vi "Variable@Range__Parameter.vi"(1 "ParamterIn":string) -> (0 "ParamterOut":string)   [LabVIEW 2019]
panel:
  in  "ParameterDst":string(combo)
  in  "End":string(combo)
  in  "Section":string(combo)
  in  "Start":string(combo)
  in  "ParameterName":string(combo)
  in  "Confirm":bool
  # "Variable@Range $VariableDst,$VariableSrc,$Start,$End(,$Section)\n          aa  bb  cc  dd  ee  ff  gg  hh\n Start   0    1    2   3   4    5   6   7\n End    -8  -7   -6  -5  -4  -3  -2  -1 \nVariable@Range $VariableDst,$VariableSrc,$Start,+$Length(,$Section)\n                         Var1,Var2,0,+2\nIf $Start is Null, $Start is 0\nIf $End is Null, $End is -1"
  # "~"
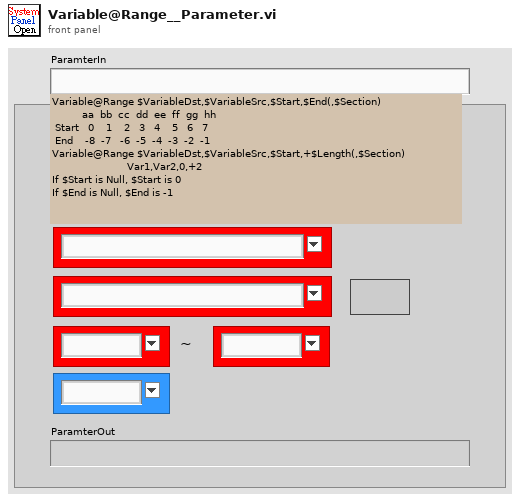
[diagram p1: front panel]
types:
  T1 = enum16{"Get", "Init", "Set", "Delete", "GetElement", "Inc", "Dec", "ReName"}
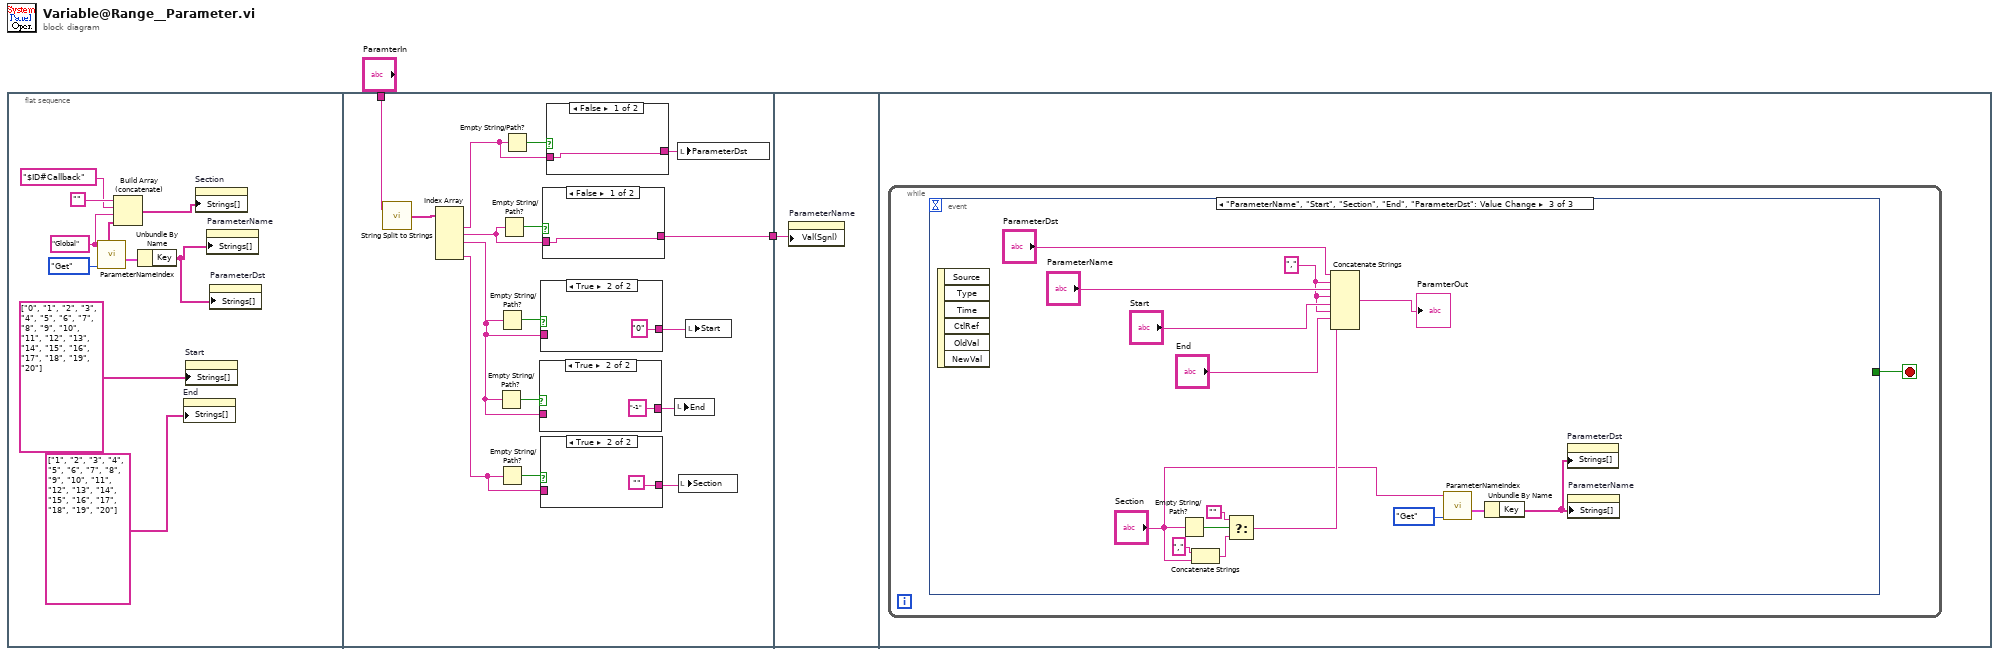
[diagram p0: block diagram]
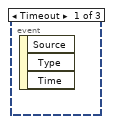
[diagram p7: hidden frame]
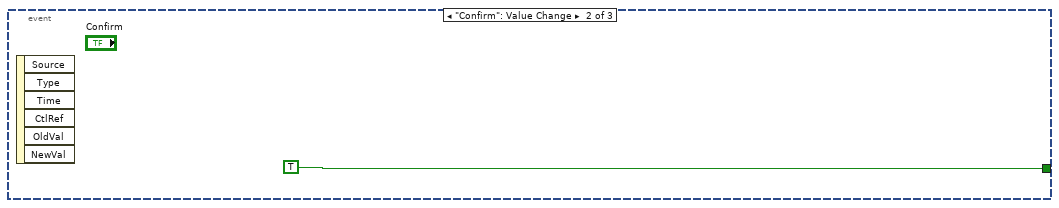
[diagram p8: hidden frame]
diagram:
  n1 = flat-sequence {
    tunnel: "ParamterIn" -> [w24]
    tunnel: [w26] -> w1
    tunnel: w1 -> [w39]
    frame #0 {
      w5 = "Global" ("VariableSection")
      n2 = call "ParameterNameIndex.vi"("OP"=T1."Get", "VariableSection"=w5) -> ("GlobalKeyValue"=w12:cluster{"Key":string[], "Value":string[]}, "SectionList"=w6:string[])  [unwired: 3 in, 5 out]
      n3 = Build Array (concatenate)("", "$ID#Callback" ("VariableSection"), w5, w6) -> (w4:string[])
      n4 = Unbundle By Name(w12) -> ("Key"=w8:string[])
      n5 = property on="End" class="CmbBox"("Strings[]"=string[] ["1", "2", "3", "4", "5", "6", "7", "8", "9", "10", "11", "12", "13", "14", "15", "16", "17", "18", "19", "20"] ("Strings []")) -> ()  [unwired: 2 in, 2 out]
      n6 = property on="Start" class="CmbBox"("Strings[]"=string[] ["0", "1", "2", "3", "4", "5", "6", "7", "8", "9", "10", "11", "12", "13", "14", "15", "16", "17", "18", "19", "20"] ("Strings []")) -> ()  [unwired: 2 in, 2 out]
      n7 = property on="Section" class="CmbBox"("Strings[]"=w4) -> ()  [unwired: 2 in, 2 out]
      n8 = property on="ParameterName" class="CmbBox"("Strings[]"=w8) -> ()  [unwired: 2 in, 2 out]
      n9 = property on="ParameterDst" class="CmbBox"("Strings[]"=w8) -> ()  [unwired: 2 in, 2 out]
    }
    frame #1 {
      n10 = call "String Split to Strings.vi"("String"=w24) -> ("Array"=w23:string[])  [unwired: 1 in]
      n11 = Index Array(array=w23) -> (element #1=w14:string, element #2=w22:string, element #3=w17:string, element #5=w19:string)  [unwired: 5 in, 1 out]
      n12 = Empty String/Path?(string/path=w17) -> (empty?=w18:bool)
      n13 = Empty String/Path?(string/path=w17) -> (empty?=w27:bool)
      n14 = Empty String/Path?(string/path=w19) -> (empty?=w21:bool)
      n15 = Empty String/Path?(string/path=w22) -> (empty?=w28:bool)
      n16 = Empty String/Path?(string/path=w14) -> (empty?=w15:bool)
      n17 = case shown="True" w18 {
        tunnel: w17 -> [w31 _]
        tunnel: [w31 "-1"] -> w16
        frame False {
        }
        frame True {
        }
      }
      n18 = case shown="True" w27 {
        tunnel: w17 -> [w35 _]
        tunnel: [w35 "0"] -> w25
        frame False {
        }
        frame True {
        }
      }
      n19 = case shown="True" w21 {
        tunnel: w19 -> [w33 _]
        tunnel: [w33 ""] -> w20
        frame False {
        }
        frame True {
        }
      }
      n20 = case shown="False" w28 {
        tunnel: w22 -> [w37 w38]
        tunnel: [w37 w38] -> w26
        frame False {
        }
        frame True {
        }
      }
      n21 = case shown="False" w15 {
        tunnel: w14 -> [w29 w30]
        tunnel: [w29 w30] -> w13
        frame False {
        }
        frame True {
        }
      }
      n22 = local write "End"(w16) -> ()
      n23 = local write "ParameterDst"(w13) -> ()
      n24 = local write "Section"(w20) -> ()
      n25 = local write "Start"(w25) -> ()
    }
    frame #2 {
      n26 = property on="ParameterName" class="CmbBox"("Val(Sgnl)"=w39) -> ()  [unwired: 2 in, 2 out]
    }
    frame #3 {
      n27 = while {
        stop <- w40 stop-if-true
        n28 = event shown="[2] \"ParameterName\", \"Start\", \"Section\", \"End\", \"ParameterDst\": Value Change" {
          selector: _ -> [_ _ _]
          dyn-events: _ -> [_ _ _]
          timeout: _ -> [_ _ _]
          tunnel: [_ TRUE _] -> w40
          event Timeout {
            n29 = event-data() -> ()  [unwired: 1 in, 3 out]
          }
          event "Confirm": Value Change {
            n30 = event-data() -> ()  [unwired: 1 in, 6 out]
          }
          event "ParameterName", "Start", "Section", "End", "ParameterDst": Value Change {
            w47 = "," ("string")
            n31 = event-data() -> ()  [unwired: 1 in, 6 out]
            n32 = Empty String/Path?(string/path="Section") -> (empty?=w52:bool)
            n33 = Concatenate Strings("," ("string"), "Section") -> (w53:string)
            n34 = Select(t="", s=w52, f=w53) -> (s? t:f=w48:string)
            n35 = Concatenate Strings("ParameterDst", w47, "ParameterName", w47, "Start", w47, "End", w48) -> (→"ParamterOut":string)
            n36 = call "ParameterNameIndex.vi"("OP"=T1."Get", "VariableSection"="Section") -> ("GlobalKeyValue"=w43:cluster{"Key":string[], "Value":string[]})  [unwired: 3 in, 6 out]
            n37 = Unbundle By Name(w43) -> ("Key"=w45:string[])
            n38 = property on="ParameterDst" class="CmbBox"("Strings[]"=w45) -> ()  [unwired: 2 in, 2 out]
            n39 = property on="ParameterName" class="CmbBox"("Strings[]"=w45) -> ()  [unwired: 2 in, 2 out]
          }
        }
      }
    }
  }
